vi "Add .NET Event Registration.vi"(10 "Event Callback Refnum":refnum<k27>, 11 "SourceGrid in":refnum<class "SourceGrid.lvclass">) -> (3 "SourceGrid out":refnum<class "SourceGrid.lvclass">)   [LabVIEW 2024, in "SourceGrid.lvlib" / "SourceGrid.lvclass"]
uses:
  SourceGrid.lvclass/SourceGrid.ctl
  SourceGrid.lvclass
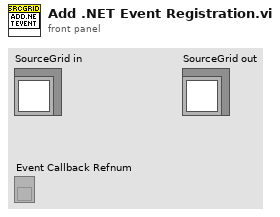
[diagram p1: front panel]
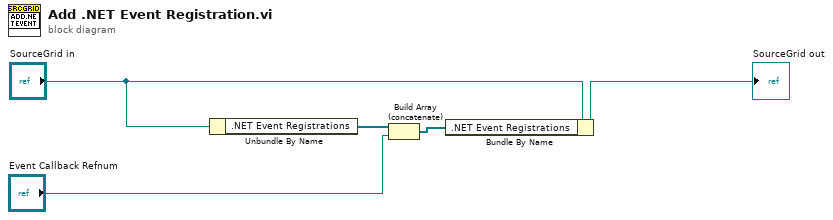
[diagram p0: block diagram]
diagram:
  n1 = Unbundle By Name("SourceGrid in") -> (".NET Event Registrations"=w3:refnum<k27>[])
  n2 = Build Array (concatenate)(w3, "Event Callback Refnum") -> (w2:refnum<k27>[])
  n3 = Bundle By Name(cluster="SourceGrid in", ".NET Event Registrations"=w2) -> (→"SourceGrid out":refnum<class "SourceGrid.lvclass">)
